vi "Register.vi"(8 "error in (no error)":errorcluster) -> (0 "error out":errorcluster)   [LabVIEW 2019, in "Camera Engine.lvlib"]
uses:
  Camera Engine.lvlib
panel:
  # "Input"
  # "Output"
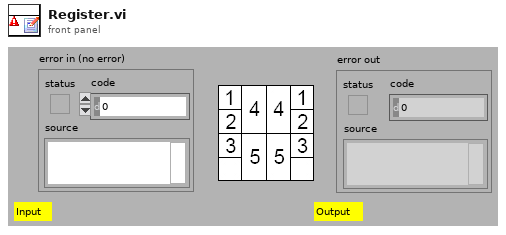
[diagram p1: front panel]
types:
  T1 = typedef "Event Message.lvlib/Event.ctl" = refnum<user-event>
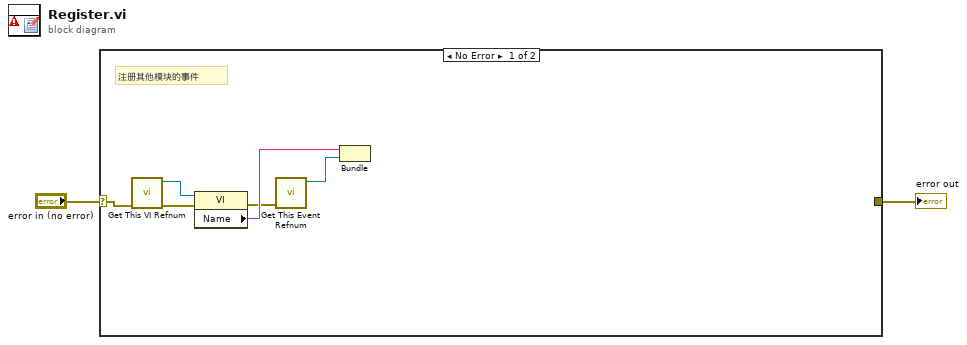
[diagram p0: block diagram]
diagram:
  n1 = case shown="No Error" "error in (no error)" {
    selector: "error in (no error)" -> [w5 w9]
    tunnel: [_ w9] -> w1
    frame No Error {
      # "注册其他模块的事件"
      n2 = call "Get This VI Refnum.vi"("error in (no error)"=w5) -> ("error out"=w4:errorcluster, "This VI Refnum Out"=w6:refnum<vi>)  [unwired: 9 in]
      n3 = property class="VI"(reference=w6, error in=w4) -> (error out=w3:errorcluster, "Name"=w7:string)  [unwired: 1 out]
      n4 = call "Get This Event Refnum.vi"("error in (no error)"=w3) -> ("This Event Refnum Out"=w8:T1)  [unwired: 9 in, 1 out]
      n5 = Bundle("Name"=w7, "This Event Refnum Out"=w8) -> ()  [unwired: 1 in, 1 out]
    }
    frame Error {
    }
  }
  "error out" <- w1
